vi "Handle getAll.vi"(8 "error in (no error)":errorcluster, 11 "RP100 in":refnum<class "RP100.lvclass">) -> (0 "error out":errorcluster, 2 "getAll":variant, 3 "RP100 out":refnum<class "RP100.lvclass">)   [LabVIEW 2019, in "RP100.lvclass"]
uses:
  RP100.lvclass
  Typedefs/Output Channel--Enum.ctl
  RP100.lvclass/RP100.ctl
  <userlib>/LevyLab/AH2500A/SMOs/AH2500A/AH2500A.lvclass
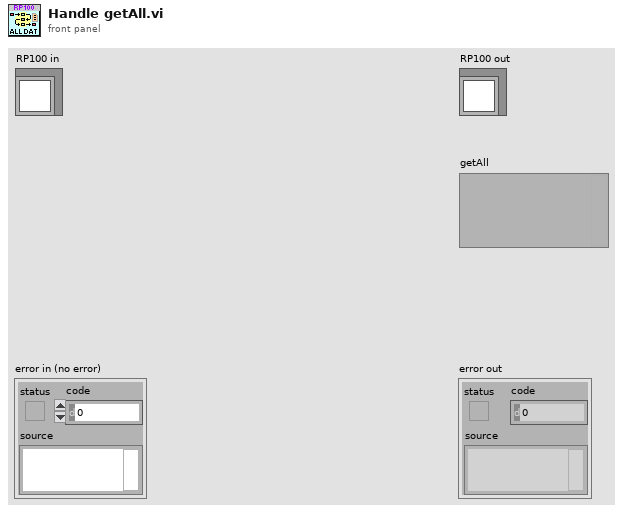
[diagram p1: front panel]
types:
  T1 = typedef "RP100.lvclass/Output Channel--Enum.ctl" = enum16{"Output 1", "Output 2"}
  T2 = typedef "RP100.lvclass/Output State--Enum.ctl" = enum16{"Shorted", "Enabled"}
  T3 = typedef "AH2500A.lvclass/AH2500A Measurement--Cluster.ctl" = cluster{"capacitance (pF)":dbl, "loss (nS)":dbl, "Vexc (V)":dbl}
  T4 = typedef "RP100.lvclass/getAll.ctl" = cluster{"Output State Ch1":string, "Output State Ch2":string, "Level (V) Ch1":dbl, "Level (V) Ch2":dbl, "Slew (V/s) Ch1":dbl, "Slew (V/s) Ch2":dbl, "measured V (V) Ch1":dbl, "measured V (V) Ch2":dbl, "measured I (A) Ch1":dbl, "measured I (A) Ch2":dbl, "bridge C (pF)":dbl, "bridge Loss (nS)":dbl, "bridge exc (V)":dbl}
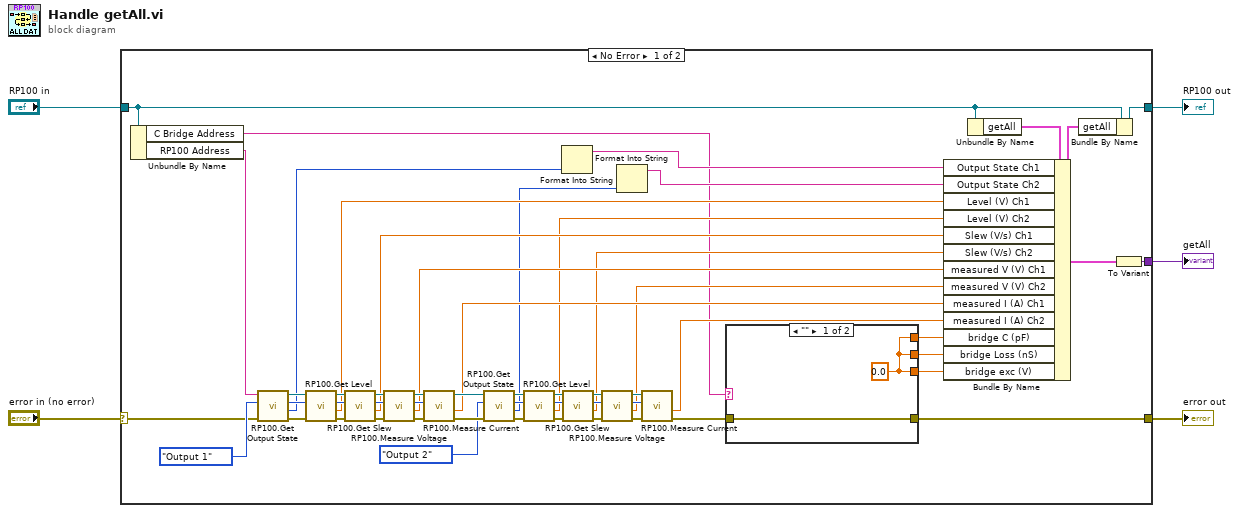
[diagram p0: block diagram]
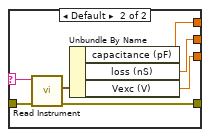
[diagram p2: hidden frame]
diagram:
  n1 = case shown="No Error" "error in (no error)" {
    selector: "error in (no error)" -> [w12 w69]
    tunnel: [w9 w69] -> w4
    tunnel: [w21 w68] -> w3
    tunnel: "RP100 in" -> [w13 w68]
    tunnel: [w19 _] -> w1
    frame No Error {
      n2 = Unbundle By Name(w13) -> ("C Bridge Address"=w10:string, "RP100 Address"=w14:string)
      n3 = call "RP100.Get Output State.vi"("error in (no error)"=w12, "Output Channel"=Output_Channel--Enum."Output 1", "VISA resource name"=w14) -> ("error out"=w47:errorcluster, "Output State"=w18:T2, "Output Channel"=w36:T1, "VISA Refnum out"=w48:refnum<visa-resource-name>)  [unwired: 5 in]
      n4 = call "RP100.Get Level.vi"("error in (no error)"=w47, "Output Channel"=w36, "VISA resource name"=w48) -> ("error out"=w45:errorcluster, "Level (V)"=w30:dbl, "Output Channel"=w35:T1, "VISA Refnum out"=w46:refnum<visa-resource-name>)  [unwired: 5 in]
      n5 = call "RP100.Get Slew.vi"("error in (no error)"=w45, "Output Channel"=w35, "VISA resource name"=w46) -> ("error out"=w43:errorcluster, "Slew (V/s)"=w29:dbl, "Output Channel"=w34:T1, "VISA Refnum out"=w44:refnum<visa-resource-name>)  [unwired: 5 in]
      n6 = call "RP100.Measure Voltage.vi"("error in (no error)"=w43, "Output"=w34, "VISA resource name"=w44) -> ("error out"=w57:errorcluster, "measured V"=w28:dbl, "Output"=w56:T1, "VISA Refnum out"=w58:refnum<visa-resource-name>)  [unwired: 5 in]
      n7 = call "RP100.Measure Current.vi"("error in (no error)"=w57, "Output Channel"=w56, "VISA resource name"=w58) -> ("error out"=w52:errorcluster, "measured I"=w27:dbl, "VISA Refnum out"=w51:refnum<visa-resource-name>)  [unwired: 5 in, 1 out]
      n8 = call "RP100.Get Output State.vi"("error in (no error)"=w52, "Output Channel"=Output_Channel--Enum."Output 2", "VISA resource name"=w51) -> ("error out"=w41:errorcluster, "Output State"=w16:T2, "Output Channel"=w33:T1, "VISA Refnum out"=w42:refnum<visa-resource-name>)  [unwired: 5 in]
      n9 = call "RP100.Get Level.vi"("error in (no error)"=w41, "Output Channel"=w33, "VISA resource name"=w42) -> ("error out"=w39:errorcluster, "Level (V)"=w26:dbl, "Output Channel"=w32:T1, "VISA Refnum out"=w40:refnum<visa-resource-name>)  [unwired: 5 in]
      n10 = Format Into String(w18) -> (resulting string=w17:string)  [unwired: 3 in, 1 out]
      n11 = call "RP100.Get Slew.vi"("error in (no error)"=w39, "Output Channel"=w32, "VISA resource name"=w40) -> ("error out"=w37:errorcluster, "Slew (V/s)"=w25:dbl, "Output Channel"=w31:T1, "VISA Refnum out"=w38:refnum<visa-resource-name>)  [unwired: 5 in]
      n12 = call "RP100.Measure Voltage.vi"("error in (no error)"=w37, "Output"=w31, "VISA resource name"=w38) -> ("error out"=w54:errorcluster, "measured V"=w24:dbl, "Output"=w55:T1, "VISA Refnum out"=w53:refnum<visa-resource-name>)  [unwired: 5 in]
      n13 = Format Into String(w16) -> (resulting string=w15:string)  [unwired: 3 in, 1 out]
      n14 = call "RP100.Measure Current.vi"("error in (no error)"=w54, "Output Channel"=w55, "VISA resource name"=w53) -> ("error out"=w11:errorcluster, "measured I"=w23:dbl)  [unwired: 5 in, 2 out]
      n15 = case shown="\"\"" w10 {
        selector: w10 -> [_ w66]
        tunnel: w11 -> [w60 w67]
        tunnel: [w60 w64] -> w9
        tunnel: [w59 w62] -> w8
        tunnel: [w59 w63] -> w7
        tunnel: [w59 w61] -> w6
        frame "" {
          w59 = 0.0 ("capacitance")
        }
        frame Default {
          n16 = call <userlib>:"Read Instrument.vi"("error in (no error)"=w67, "VISA resource name"=w66) -> ("error out"=w64:errorcluster, "Measurement"=w65:T3)  [unwired: 7 in, 1 out]
          n17 = Unbundle By Name(w65) -> ("capacitance (pF)"=w62:dbl, "loss (nS)"=w63:dbl, "Vexc (V)"=w61:dbl)
        }
      }
      n18 = Unbundle By Name(w13) -> ("getAll"=w22:T4)
      n19 = Bundle By Name(cluster=w22, "Output State Ch1"=w17, "Output State Ch2"=w15, "Level (V) Ch1"=w30, "Level (V) Ch2"=w26, "Slew (V/s) Ch1"=w29, "Slew (V/s) Ch2"=w25, "measured V (V) Ch1"=w28, "measured V (V) Ch2"=w24, "measured I (A) Ch1"=w27, "measured I (A) Ch2"=w23, "bridge C (pF)"=w8, "bridge Loss (nS)"=w7, "bridge exc (V)"=w6) -> (w20:T4)
      n20 = Bundle By Name(cluster=w13, "getAll"=w20) -> (w21:refnum<class "RP100.lvclass">)
      n21 = To Variant(anything=w20) -> (Variant=w19:variant)
    }
    frame Error {
    }
  }
  "error out" <- w4
  "RP100 out" <- w3
  "getAll" <- w1
